vi "5.7.4-OCU-to-Forebrain-UDPClient.vi"() -> ()   [LabVIEW 2010]
doc: "This VI implements a client for the Named Service UDP Server.vi.\nIt connects to a service by specifying the server address and the name of the service. After sending a 'Hello' string to the server, the client receives the string sent by the server, displays the string and closes the connection.\n\n<b>Note:</b> This VI is built to work with the Named Service UDP Server.vi in UDP.llb."
uses:
  6-OCU Neurons/MainControls.ctl
  6-OCU Neurons/6.1-UDP Saitek.ctl
  5.0-Global.vi
panel:
  out "address":u32
  out "port":u16
  out "Main Controls":T1 {"6.1-Saitek Controller"."Right" scale=-32767.0..32767.0; "6.1-Saitek Controller"."Left" scale=-32767.0..32767.0; "6.1-Saitek Controller"."Yaw" scale=-32767.0..32767.0; "6.1-Saitek Controller"."Roll" scale=-32767.0..32767.0; "6.1-Saitek Controller"."Pitch" scale=-32767.0..32767.0}
  out "String":string
  out "error out":errorcluster
  in  "error in":errorcluster
  # "Instructions:\n1. Open Named Service UDP Server.vi located in the same library.\n2. Follow the instructions on it's front panel.\n\nNote: This VI is built to work with the Named Service UDP Server.vi in UDP.llb."
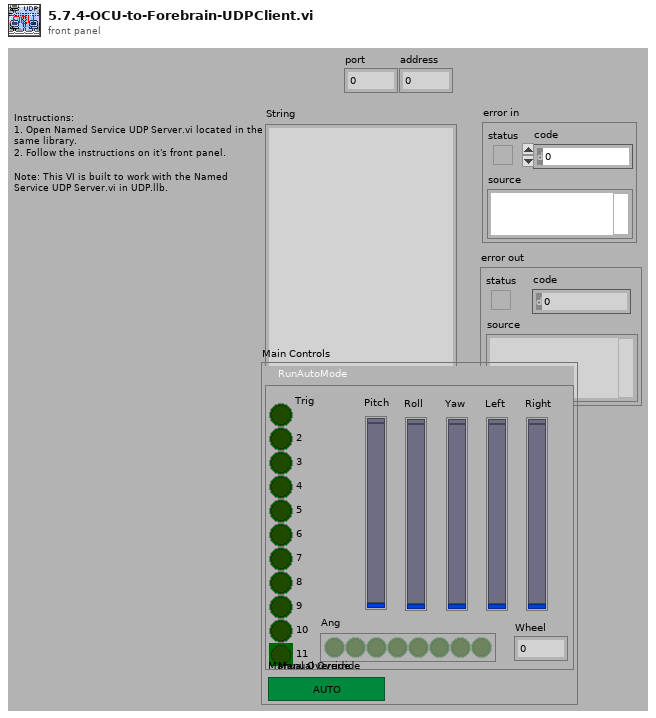
[diagram p1: front panel]
types:
  T1 = typedef "MainControls.ctl" = cluster{"6.1-Saitek Controller":T2, "Manual Override":bool}
  T2 = typedef "6.1-UDP Saitek.ctl" = cluster{"Trig":bool, "2":bool, "3":bool, "4":bool, "5":bool, "6":bool, "7":bool, "8":bool, "9":bool, "10":bool, "11":bool, "Pitch":i32, "Ang":bool[], "Wheel":dbl, "Roll":i32, "Yaw":i32, "Left":i32, "Right":i32}
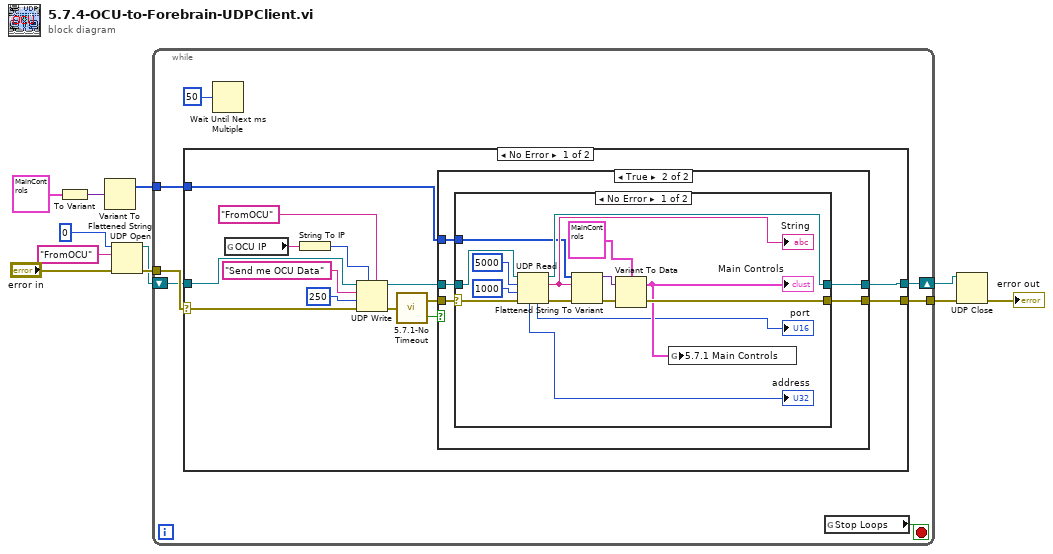
[diagram p0: block diagram]
diagram:
  n1 = To Variant(anything=T1 {"6.1-Saitek Controller"={"Trig"=FALSE, "2"=FALSE, "3"=FALSE, "4"=FALSE, "5"=FALSE, "6"=FALSE, "7"=FALSE, "8"=FALSE, "9"=FALSE, "10"=FALSE, "11"=FALSE, "Pitch"=0, "Ang"=[], "Wheel"=0.0, "Roll"=0, "Yaw"=0, "Left"=0, "Right"=0}, "Manual Override"=FALSE} ("AutoModeDatums")) -> (Variant=w5:variant)
  n2 = Variant To Flattened String(Variant=w5) -> (1:w4:i16[])  [unwired: 1 out]
  n3 = UDP Open(8:"error in", 10:"FromOCU" ("service name"), 11:u16 0 ("port")) -> (port=w9:refnum<k16>, 0:w10:errorcluster)  [unwired: 2 in, 1 out]
  n4 = while {
    tunnel: [w18] -> w7
    tunnel: w10 -> [w17]
    shift-right: [w15] -> w8
    shift-left: w9 -> [w16]
    tunnel: w4 -> [w13]
    stop <- w12 stop-if-true
    n5 = case shown="No Error" w17 {
      selector: w17 -> [w32 w58]
      tunnel: [w27 w58] -> w18
      tunnel: w16 -> [w31 w57]
      tunnel: [w26 w57] -> w15
      tunnel: w13 -> [w21 _]
      frame No Error {
        n6 = global read "5.0-Global.vi" "OCU IP"() -> (w20:string)
        n7 = String To IP(1:w20) -> (0:w30:u32)
        n8 = UDP Write(address=w30, port or service name="FromOCU", connection ID=w31, data in="Send me OCU Data", 8:w32, 9:250 ("timeout ms (25000)")) -> (error out=w25:errorcluster, 3:w28:refnum<k16>)
        n9 = call "5.7.1-No Timeout.vi"("error in (no error)"=w25) -> ("No Timeout"=w23:bool, "error out"=w24:errorcluster)
        n10 = case shown="True" w23 {
          tunnel: w24 -> [w34 w39]
          tunnel: w28 -> [w33 w38]
          tunnel: [w33 w37] -> w26
          tunnel: [w34 w36] -> w27
          tunnel: w21 -> [_ w35]
          frame False {
          }
          frame True {
            n11 = case shown="No Error" w39 {
              selector: w39 -> [w54 w55]
              tunnel: w38 -> [w53 w56]
              tunnel: [w51 w56] -> w37
              tunnel: [w44 w55] -> w36
              tunnel: w35 -> [w48 _]
              frame No Error {
                n12 = UDP Read(connection ID=w53, max size (548)=5000, timeout ms (25000)=1000, 8:w54) -> (data out=w49:string, error out=w45:errorcluster, 3:w51:refnum<k16>, 4:→"port":u16, 6:→"address":u32)
                "String" <- w49
                n13 = Flattened String To Variant(4:w45, 6:w49, 7:w48) -> (0:w46:errorcluster, 3:w47:variant)
                n14 = Variant To Data(error in=w46, Variant=w47, type=T1 {"6.1-Saitek Controller"={"Trig"=FALSE, "2"=FALSE, "3"=FALSE, "4"=FALSE, "5"=FALSE, "6"=FALSE, "7"=FALSE, "8"=FALSE, "9"=FALSE, "10"=FALSE, "11"=FALSE, "Pitch"=0, "Ang"=[], "Wheel"=0.0, "Roll"=0, "Yaw"=0, "Left"=0, "Right"=0}, "Manual Override"=FALSE} ("AutoModeDatums")) -> (error out=w44:errorcluster, data=w42:T1)
                "Main Controls" <- w42
                n15 = global write "5.0-Global.vi" "5.7.1 Main Controls"(w42) -> ()
              }
              frame Error {
              }
            }
          }
        }
      }
      frame Error {
      }
    }
    n16 = Wait Until Next ms Multiple(millisecond multiple=u32 50) -> ()  [unwired: 1 out]
    n17 = global read "5.0-Global.vi" "Stop Loops"() -> (w12:bool)
  }
  n18 = UDP Close(connection ID=w8, 8:w7) -> (error out=→"error out":errorcluster)  [unwired: 1 out]
